vi "F to K(2D dbl).vi"(1 "F":dbl[][](array[numeric])) -> (0 "K":dbl[][](array[numeric]))   [LabVIEW 2012, in "Temp Converter.lvlib"]
doc: "<B>输入端子C</B>: 输入华氏温度。\n<B>输出端子C</B>: 输出摄氏温度。\n\n公式：F-->C-->K\n创建者：CSXCS_366"
uses:
  Temp Converter.lvlib
  FtoC/F to C (2D dbl).vi
  CtoK/C to K (2D dbl).vi
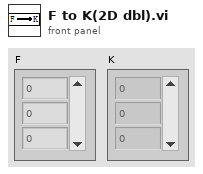
[diagram p1: front panel]
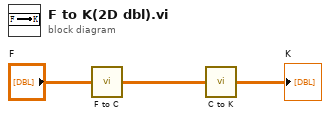
[diagram p0: block diagram]
diagram:
  n1 = call-poly "F to C.vi"("F"="F") -> ("C"=w2:dbl[][])
  n2 = call-poly "C to K.vi"("C"=w2) -> ("K"=→"K":dbl[][])
